vi "ObtainBroadcastEvents.vi"(8 "error in (no error)":errorcluster, 10 "CreateNew? (F)":bool) -> (0 "error out":errorcluster, 2 "clBroadcastEvents":T1)   [LabVIEW 2018, in "SensorShared.lvlib"]
uses:
  SensorShared.lvlib
  clBroadcastEvents.ctl
  clEventType.ctl
panel:
  # "These are the default\nBroadcast Events\nfor the cloneable module\n\nIf you want to add your own,create the typedefs in the PublicAPI/Arguments/Broadcast foldr and add event references to the clBroadcastEvents typedef in the Private/Broadcast folder."
  # "If you want to add other Broadcast Events, open this typedef, copy an existing event and rename it to your event name.\n\nNext create an \"arg\" typedef for the  data and put it into PublicAPI/Arguments/Broadcasts\n\nAfter that, you will need to create a new roadcast vi in Protected/Broadcast.  Look at DidInit.vi or the reportError.vi as examples."
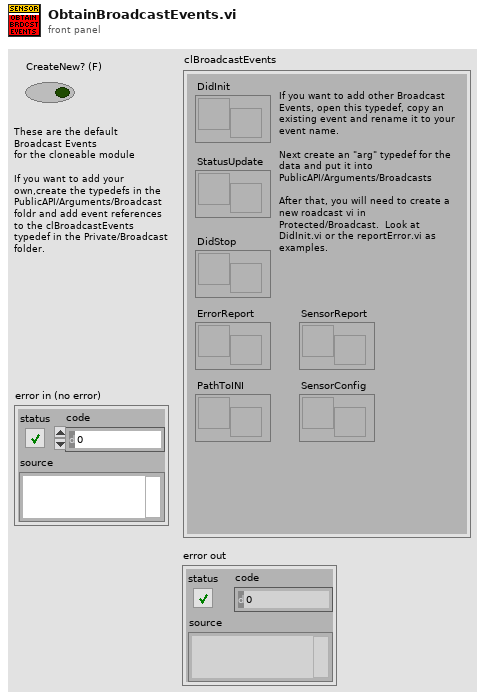
[diagram p1: front panel]
types:
  T1 = typedef "SensorShared.lvlib/clBroadcastEvents.ctl" = cluster{"DidInit":refnum<user-event>, "StatusUpdate":refnum<user-event>, "ErrorReport":refnum<user-event>, "DidStop":refnum<user-event>, "PathToINI":refnum<user-event>, "SensorReport":refnum<user-event>, "SensorConfig":refnum<user-event>}
  T2 = typedef "SensorModule.lvlib/clBroadcastEvents.ctl" = cluster{"DidInit":refnum<user-event>, "StatusUpdate":refnum<user-event>, "ErrorReport":refnum<user-event>, "DidStop":refnum<user-event>, "PathToINI":refnum<user-event>, "SensorReport":refnum<user-event>, "SensorConfig":refnum<user-event>}
  T3 = typedef "SensorShared.lvlib/clEventType.ctl" = cluster{"ModuleID":i32, "Data":variant}
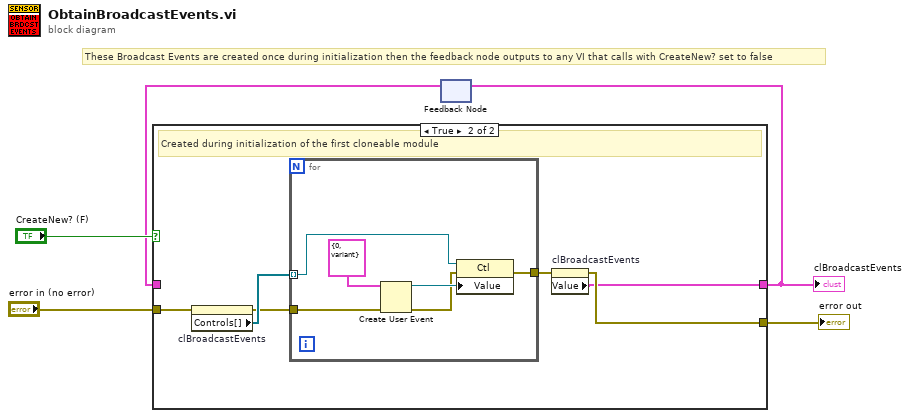
[diagram p0: block diagram]
diagram:
  # "These Broadcast Events are created once during initialization then the feedback node outputs to any VI that calls with CreateNew? set to false"
  n1 = feedback #1() -> (w2:T2)  [unwired: 1 in]
  n2 = case shown="True" "CreateNew? (F)" {
    tunnel: "error in (no error)" -> [w6 w9]
    tunnel: [w6 w13] -> w4
    tunnel: [w7 w12] -> w1
    tunnel: w2 -> [w7 _]
    frame False {
      # "Modules can register to receive these broadcasts or subesquenc cloneable modules can get the events here"
    }
    frame True {
      # "Created during initialization of the first cloneable module"
      n3 = property on="clBroadcastEvents" class="Clust (strict)"(error in=w9) -> (error out=w8:errorcluster, "Controls[]"=w10:refnum<vi>[])  [unwired: 1 in, 1 out]
      n4 = for {
        tunnel: w10 -> [w14] mode=indexing
        tunnel: w8 -> [w19]
        tunnel: [w17] -> w11
        n5 = Create User Event(user event datatype=T3 {"ModuleID"=0, "Data"=variant} ("clBroadcast"), error in=w19) -> (user event=w18:refnum<user-event>, error out=w16:errorcluster)
        n6 = property class="Ctl"(reference=w14, error in=w16, "Value"=w18) -> (error out=w17:errorcluster)  [unwired: 1 out]
      }
      n7 = property on="clBroadcastEvents" class="Clust (strict)"(error in=w11) -> (error out=w13:errorcluster, "Value"=w12:T2)  [unwired: 1 in, 1 out]
    }
  }
  "error out" <- w4
  "clBroadcastEvents" <- w1
  n8 = feedback-in #1(w1) -> ()
